vi "Transfer Settings.vi"(7 "QRD":T1, 8 "error in":errorcluster) -> (0 "error out":errorcluster, 5 "QRD Out":T1)   [LabVIEW 2025]
uses:
  Builds/Queue Wrappers.lvlibp
  Builds/Queue Wrappers.lvlibp/Q Packet.ctl
  Controls/Queues-Refs-Data.ctl
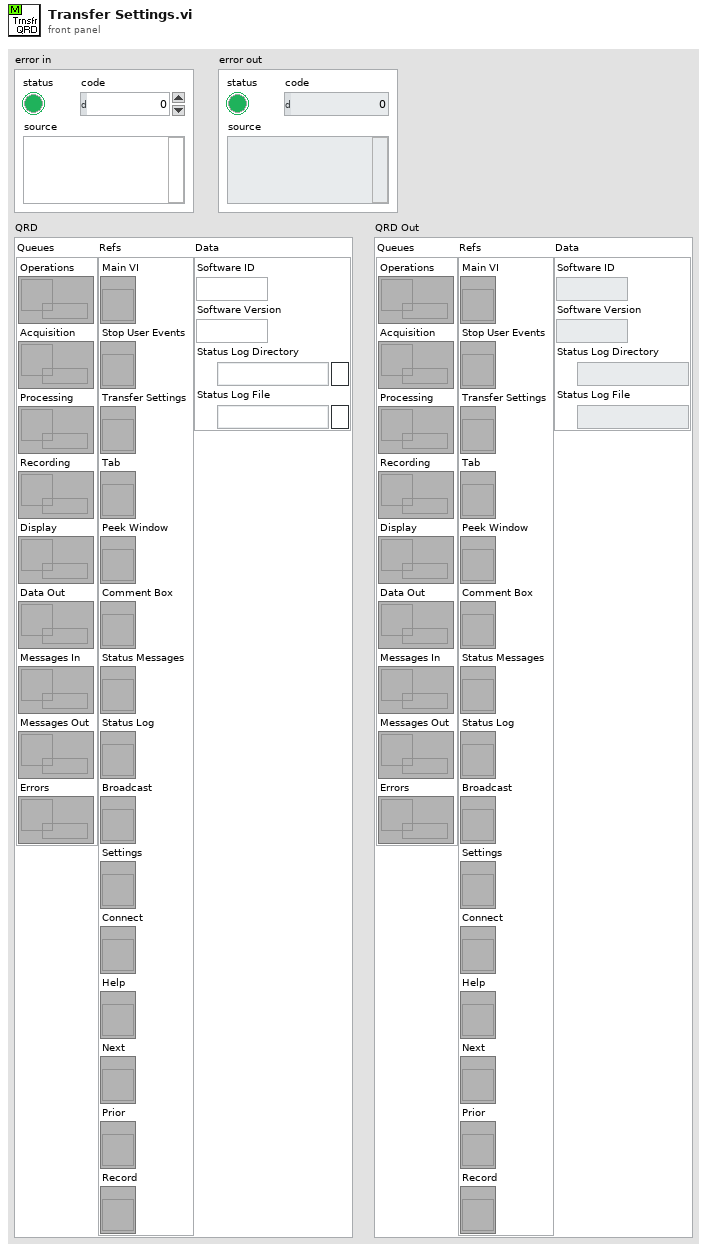
[diagram p1: front panel]
types:
  T1 = typedef "Queues-Refs-Data.ctl" = cluster{"Queues":cluster{"Operations":refnum<queue>, "Acquisition":refnum<queue>, "Processing":refnum<queue>, "Recording":refnum<queue>, "Display":refnum<queue>, "Data Out":refnum<queue>, "Messages In":refnum<queue>, "Messages Out":refnum<queue>, "Errors":refnum<queue>}, "Refs":cluster{"Main VI":refnum<vi>, "Stop User Events":refnum<vi>, "Transfer Settings":refnum<vi>, "Tab":refnum<vi>, "Peek Window":refnum<vi>, "Comment Box":refnum<vi>, "Status Messages":refnum<vi>, "Status Log":refnum<vi>, "Broadcast":refnum<vi>, "Settings":refnum<vi>, "Connect":refnum<vi>, "Help":refnum<vi>, "Next":refnum<vi>, "Prior":refnum<vi>, "Record":refnum<vi>}, "Data":cluster{"Software ID":string, "Software Version":string, "Status Log Directory":path, "Status Log File":path}}
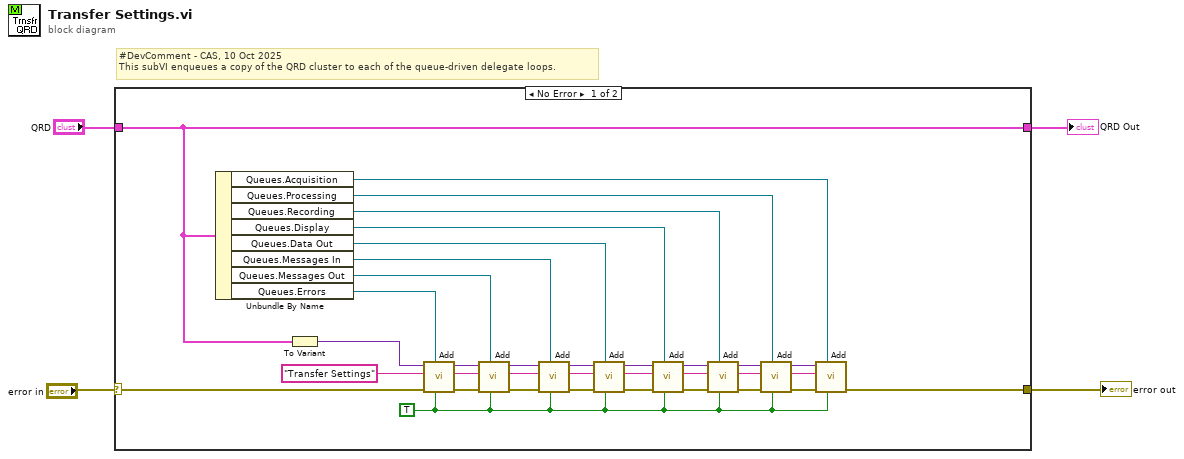
[diagram p0: block diagram]
diagram:
  # "#DevComment - CAS, 10 Oct 2025\nThis subVI enqueues a copy of the QRD cluster to each of the queue-driven delegate loops."
  n1 = case shown="No Error" "error in" {
    selector: "error in" -> [w39 w41]
    tunnel: [w21 w40] -> w4
    tunnel: "QRD" -> [w21 w40]
    tunnel: [w23 w41] -> w2
    frame No Error {
      w22 = TRUE ("Priority Message")
      n2 = Unbundle By Name(w21) -> ("Queues.Acquisition"=w24:refnum<queue>, "Queues.Processing"=w25:refnum<queue>, "Queues.Recording"=w26:refnum<queue>, "Queues.Display"=w27:refnum<queue>, "Queues.Data Out"=w28:refnum<queue>, "Queues.Messages In"=w29:refnum<queue>, "Queues.Messages Out"=w30:refnum<queue>, "Queues.Errors"=w38:refnum<queue>)
      n3 = To Variant(anything=w21) -> (Variant=w5:variant)
      n4 = call "Add.vi"("Priority Message"=w22, "Q Ref In"=w38, "error in"=w39, "Message ID"="Transfer Settings" ("Packet ID"), "Payload"=w5) -> ("error out"=w35:errorcluster, "Message ID Out"=w19:string, "Payload Out"=w20:variant)  [unwired: 3 in, 1 out]
      n5 = call "Add.vi"("Priority Message"=w22, "Q Ref In"=w30, "error in"=w35, "Message ID"=w19, "Payload"=w20) -> ("error out"=w34:errorcluster, "Message ID Out"=w17:string, "Payload Out"=w18:variant)  [unwired: 3 in, 1 out]
      n6 = call "Add.vi"("Priority Message"=w22, "Q Ref In"=w29, "error in"=w34, "Message ID"=w17, "Payload"=w18) -> ("error out"=w33:errorcluster, "Message ID Out"=w15:string, "Payload Out"=w16:variant)  [unwired: 3 in, 1 out]
      n7 = call "Add.vi"("Priority Message"=w22, "Q Ref In"=w28, "error in"=w33, "Message ID"=w15, "Payload"=w16) -> ("error out"=w37:errorcluster, "Message ID Out"=w13:string, "Payload Out"=w14:variant)  [unwired: 3 in, 1 out]
      n8 = call "Add.vi"("Priority Message"=w22, "Q Ref In"=w27, "error in"=w37, "Message ID"=w13, "Payload"=w14) -> ("error out"=w32:errorcluster, "Message ID Out"=w11:string, "Payload Out"=w12:variant)  [unwired: 3 in, 1 out]
      n9 = call "Add.vi"("Priority Message"=w22, "Q Ref In"=w26, "error in"=w32, "Message ID"=w11, "Payload"=w12) -> ("error out"=w36:errorcluster, "Message ID Out"=w9:string, "Payload Out"=w10:variant)  [unwired: 3 in, 1 out]
      n10 = call "Add.vi"("Priority Message"=w22, "Q Ref In"=w25, "error in"=w36, "Message ID"=w9, "Payload"=w10) -> ("error out"=w31:errorcluster, "Message ID Out"=w7:string, "Payload Out"=w8:variant)  [unwired: 3 in, 1 out]
      n11 = call "Add.vi"("Priority Message"=w22, "Q Ref In"=w24, "error in"=w31, "Message ID"=w7, "Payload"=w8) -> ("error out"=w23:errorcluster)  [unwired: 3 in, 3 out]
    }
    frame Error {
    }
  }
  "error out" <- w2
  "QRD Out" <- w4
